vi "Append tiff file strings.vi"(3 "error in":errorcluster, 4 "Tiff file (B)":string, 5 "Tiff file or stack (A)":string) -> (0 "error out":errorcluster, 1 "Merged (A+B)":string)   [LabVIEW 2015, in "Tiff reader.lvlib"]
doc: "This .vi merges a single TIF image into an exisitng TIF image or stack, to make a TIF stack."
uses:
  Tiff reader.lvlib
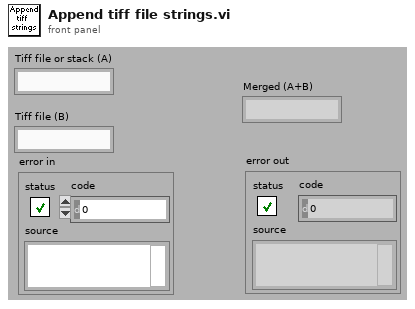
[diagram p1: front panel]
types:
  T1 = typedef "Tiff reader.lvlib/IFD Entry.ctl" = cluster{"Tag":u16, "Type":T2, "Count":u32, "Val/Offs":u32, "Is Pointer?":bool, "Byte stream index":i32}
  T2 = typedef "Tiff reader.lvlib/FieldTypes.ctl" = enum16{"NULL", "U8", "ASCII7", "U16", "U32", "RATIONAL", "SByte(I8)", "Undef(8Bit)", "I16", "I32", "SRat(4B:4B)", "SGL(4Byte)", "DBL(8Byte)"}
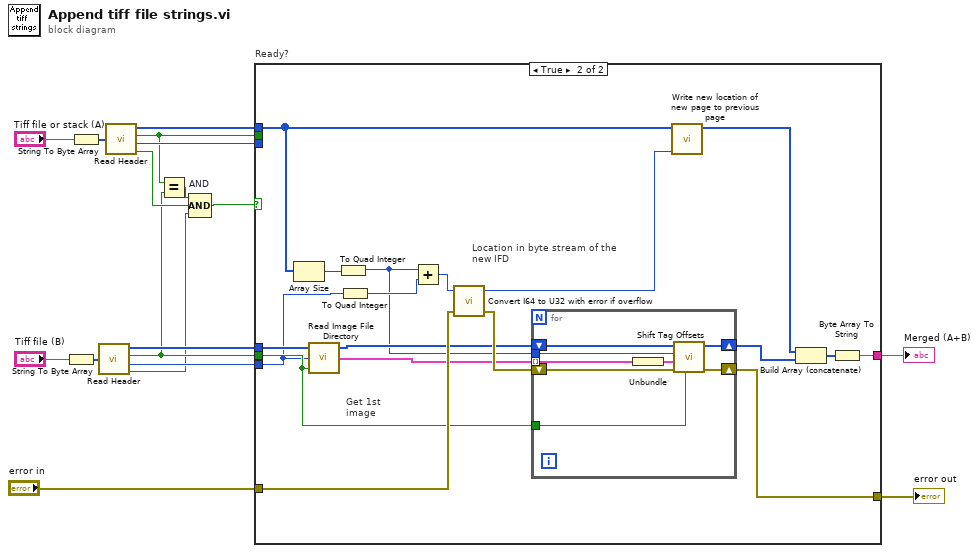
[diagram p0: block diagram]
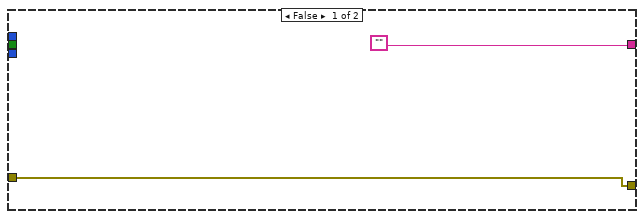
[diagram p2: hidden frame]
diagram:
  n1 = String To Byte Array(string="Tiff file (B)") -> (unsigned byte array=w15:u8[])
  n2 = String To Byte Array(string="Tiff file or stack (A)") -> (unsigned byte array=w12:u8[])
  n3 = call "Read Header.vi"("TIFF Data in"=w15) -> ("TIFF Data out"=w16:u8[], "Litt/BigEnd"=w5:bool, "ImFileDirectOffs"=w17:u32, "IsTIFF?"=w4:bool)
  n4 = call "Read Header.vi"("TIFF Data in"=w12) -> ("TIFF Data out"=w14:u8[], "Litt/BigEnd"=w6:bool, "ImFileDirectOffs"=w13:u32, "IsTIFF?"=w8:bool)
  n5 = Equal?(x=w6, y=w5) -> (x = y?=w7:bool)
  n6 = Compound Arithmetic op=AND "AND"(w7, w8, w4) -> (w3:bool)
  n7 = case "Ready?" shown="True" w3 {
    tunnel: w17 -> [_ w27]
    tunnel: w16 -> [_ w35]
    tunnel: w14 -> [_ w33]
    tunnel: w13 -> [_ _]
    tunnel: ["" w31] -> w11
    tunnel: w6 -> [_ _]
    tunnel: w5 -> [_ w28]
    tunnel: "error in" -> [w18 w37]
    tunnel: [w18 w23] -> w1
    frame False {
    }
    frame True {
      # "Location in byte stream of the \nnew IFD"
      # "Get 1st\nimage"
      n8 = Array Size(array=w33) -> (size(s)=w22:i32)
      n9 = call "Read Image File Directory.vi"("Litt/BigEnd"=w28, "Im_File_Dir Offs"=w27, "Image Data in"=w35) -> ("Directories"=w20:cluster{"Tags":T1[]}[], "Image Data out"=w30:u8[])  [unwired: 1 out]
      n10 = To Quad Integer(1:w22) -> (0:w21:i64)
      n11 = To Quad Integer(1:w27) -> (0:w26:i64)
      n12 = Add(x=w21, y=w26) -> (x+y=w25:i64)
      n13 = call "Convert I64 to U32 with error if overflow.vi"("error in"=w37, "I64"=w25) -> ("error out"=w36:errorcluster, "U32"=w24:u32)  [unwired: 2 out]
      n14 = for {
        tunnel: w28 -> [w42]
        tunnel: w21 -> [w39]
        tunnel: w20 -> [w38] mode=indexing
        shift-right: [w40] -> w23
        shift-left: w36 -> [w45]
        shift-right: [w43] -> w29
        shift-left: w30 -> [w44]
        n15 = Unbundle(w38) -> ("Tags"=w41:T1[])
        n16 = call "Shift Tag Offsets.vi"("Litt/BigEnd"=w42, "error in"=w45, "Tags"=w41, "# of bytes inserted before tag data"=w39, "Image Data"=w44) -> ("error out"=w40:errorcluster, "Image Data Out"=w43:u8[])  [unwired: 4 in, 1 out]
      }
      n17 = call "Write new location of new page to previous page.vi"("Location in byte stream of the \nnew IFD"=w24, "Image Data in"=w33) -> ("Image Data out"=w34:u8[])  [unwired: 3 in, 6 out]
      n18 = Build Array (concatenate)(w34, w29) -> (w32:u8[])
      n19 = Byte Array To String(unsigned byte array=w32) -> (string=w31:string)
    }
  }
  "Merged (A+B)" <- w11
  "error out" <- w1
